vi "FMPA LogSort_Partition.vi"(0 "Array In":string[](array[string]), 2 "Indices":cluster{"First":i32, "Last":i32}) -> (14 "Array Out":string[](array[string]), 17 "Split":i32)   [LabVIEW 2023]
doc: "The split algorithm starts by indexing the splitpoint value from subarray at the First index. It compares the split point value to all elements from index First + 1 to Last. When an smaller element is found, the splitpoint index is incremented, and its the element at the new location is swapped with the smaller element. \n\nThe splitpoint value and splitpoint index may cause some confusion. The split point value is indexed out before the For Loop begins executing, but the splitpoint index is incremented as elements are swapped. After the For Loop terminates, the elements at the First index and splitpoint are swapped. Thus, all subarray elements at locations smaller than the splitpoint index are less than the splitpoint value and all elements at higher locations are not less than the splitpoint value.\n\nPseudocode\n procedure split (first, last, splitpoint, as)\n\n x = a[first]\n\n splitpt = first\n\n for i = first + 1 to last\n\n if a[i] < x then\n\n swap (a[++splitpoint], a[i])\n\n endif\n\n endfor\n\n swap (a[first], a[splitpoint])"
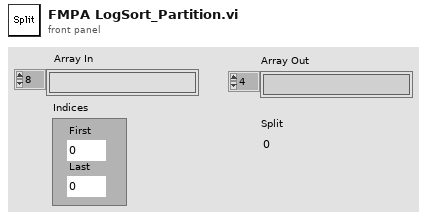
[diagram p1: front panel]
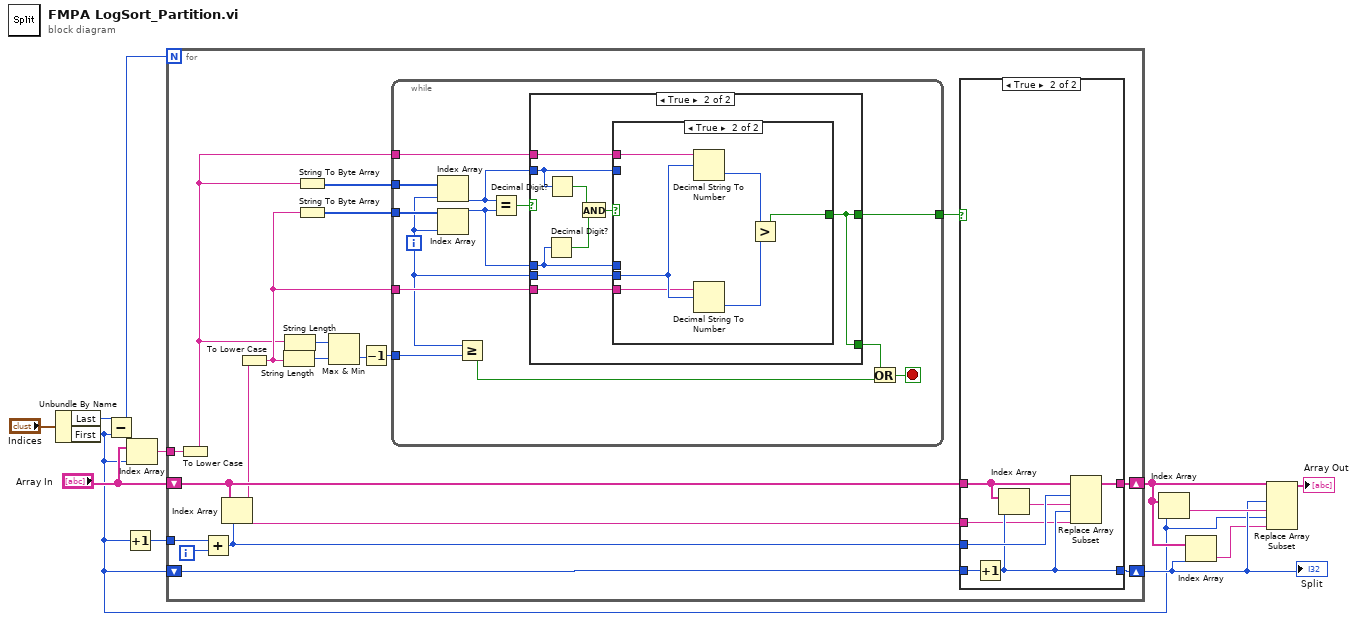
[diagram p0: block diagram]
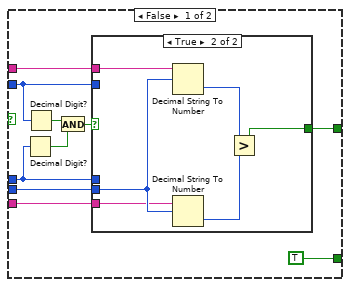
[diagram p2: hidden frame]
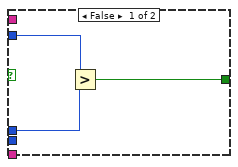
[diagram p3: hidden frame]
diagram:
  n1 = Unbundle By Name("Indices") -> ("Last"=w9:i32, "First"=w2:i32)
  n2 = Subtract(x=w9, y=w2) -> (x-y=w1:i32)
  n3 = Increment(x=w2) -> (x+1=w11:i32)
  n4 = Index Array(array="Array In", index=w2) -> (element=w12:string)
  n5 = for {
    N: w1 -> [_]
    shift-right: [w27] -> w6
    shift-left: "Array In" -> [w28]
    tunnel: w12 -> [w16]
    tunnel: w11 -> [w29]
    shift-right: [w25] -> w4
    shift-left: w2 -> [w26]
    i -> [w30]
    n6 = To Lower Case(string=w16) -> (all lower case string=w13:string)
    n7 = Add(x=w29, y=w30) -> (x+y=w24:i32)
    n8 = Index Array(array=w28, index=w24) -> (element=w14:string)
    n9 = To Lower Case(string=w14) -> (all lower case string=w21:string)
    n10 = String Length(string=w21) -> (length=w17:i32)
    n11 = String Length(string=w13) -> (length=w18:i32)
    n12 = String To Byte Array(string=w13) -> (unsigned byte array=w23:u8[])
    n13 = String To Byte Array(string=w21) -> (unsigned byte array=w22:u8[])
    n14 = Max & Min(x=w18, y=w17) -> (min(x,y)=w20:i32)  [unwired: 1 out]
    n15 = Decrement(x=w20) -> (x-1=w19:i32)
    n16 = while {
      tunnel: w23 -> [w43]
      tunnel: w22 -> [w42]
      tunnel: [w31] -> w15
      tunnel: w13 -> [w39]
      tunnel: w21 -> [w38]
      tunnel: w19 -> [w35]
      i -> [w36]
      stop <- w33 stop-if-true
      n17 = Index Array(array=w43, index=w36) -> (element=w41:u8)
      n18 = Index Array(array=w42, index=w36) -> (element=w40:u8)
      n19 = Greater Or Equal?(x=w36, y=w35) -> (x >= y?=w34:bool)
      n20 = Equal?(x=w41, y=w40) -> (x = y?=w37:bool)
      n21 = case shown="True" w37 {
        tunnel: w41 -> [w53 w71]
        tunnel: w40 -> [w52 w70]
        tunnel: w39 -> [w51 w69]
        tunnel: w38 -> [w50 w68]
        tunnel: w36 -> [w49 w67]
        tunnel: [w45 w63] -> w31
        tunnel: [TRUE w63] -> w32
        frame False {
          n22 = Decimal Digit?(1:w52) -> (0:w47:bool)
          n23 = Decimal Digit?(1:w53) -> (0:w48:bool)
          n24 = And(x=w48, y=w47) -> (x .and. y?=w46:bool)
          n25 = case shown="True" w46 {
            tunnel: w53 -> [w56 _]
            tunnel: w52 -> [w55 _]
            tunnel: [w54 w59] -> w45
            tunnel: w49 -> [_ w62]
            tunnel: w51 -> [_ w58]
            tunnel: w50 -> [_ w57]
            frame False {
              n26 = Greater?(x=w56, y=w55) -> (0:w54:bool)
            }
            frame True {
              n27 = Decimal String To Number(string=w58, offset=w62) -> (number=w61:i32)  [unwired: 1 in, 1 out]
              n28 = Decimal String To Number(string=w57, offset=w62) -> (number=w60:i32)  [unwired: 1 in, 1 out]
              n29 = Greater?(x=w61, y=w60) -> (0:w59:bool)
            }
          }
        }
        frame True {
          n30 = Decimal Digit?(1:w70) -> (0:w65:bool)
          n31 = Decimal Digit?(1:w71) -> (0:w66:bool)
          n32 = And(x=w66, y=w65) -> (x .and. y?=w64:bool)
          n33 = case shown="True" w64 {
            tunnel: w71 -> [_ _]
            tunnel: w70 -> [_ _]
            tunnel: [_ w74] -> w63
            tunnel: w67 -> [_ w77]
            tunnel: w69 -> [_ w73]
            tunnel: w68 -> [_ w72]
            frame False {
            }
            frame True {
              n34 = Decimal String To Number(string=w73, offset=w77) -> (number=w76:i32)  [unwired: 1 in, 1 out]
              n35 = Decimal String To Number(string=w72, offset=w77) -> (number=w75:i32)  [unwired: 1 in, 1 out]
              n36 = Greater?(x=w76, y=w75) -> (0:w74:bool)
            }
          }
        }
      }
      n37 = Or(x=w32, y=w34) -> (x .or. y?=w33:bool)
    }
    n38 = case shown="True" w15 {
      tunnel: w28 -> [w79 w84]
      tunnel: [w79 w85] -> w27
      tunnel: w26 -> [w78 w86]
      tunnel: [w78 w81] -> w25
      tunnel: w14 -> [_ w80]
      tunnel: w24 -> [_ w83]
      frame False {
      }
      frame True {
        n39 = Increment(x=w86) -> (x+1=w81:i32)
        n40 = Index Array(array=w84, index=w81) -> (element=w82:string)
        n41 = Replace Array Subset(array=w84, new element #1=w82, index #1=w83, new element #2=w80, index #2=w81) -> (w85:string[])
      }
    }
  }
  "Split" <- w4
  n42 = Index Array(array=w6, index=w2) -> (element=w5:string)
  n43 = Index Array(array=w6, index=w4) -> (element=w3:string)
  n44 = Replace Array Subset(array=w6, new element #1=w5, index #1=w4, new element #2=w3, index #2=w2) -> (→"Array Out":string[])
